vi "Channels.Inline.Block Data Ref to Descriptor.vi"(8 "error in (no error)":errorcluster, 11 "Block Data Ref":T3[](array[typedef]) {"Data Reference" format="%.0x"}) -> (0 "error out":errorcluster, 3 "Channel Block Descriptor":T1[](array[typedef]))   [LabVIEW 2016, in "VeriStand Data.lvlib"]
doc: "Converts a VeriStand <B>Block Data Ref</B> into a <B>Channel Block Descriptor</B> to allow for direct access of channel data."
uses:
  VeriStand Data.lvlib
  <vilib>/NI Veristand/Custom Device API/Block Data Reference.ctl
  <vilib>/NI Veristand/Custom Device API/Data Reference.ctl
  Typedefs/Typedefs.Block Descriptor.Channel Block.ctl
  Typedefs/Typedefs.Block Descriptor.ctl
  Channels.Inline.Data Reference to Pointer.vi
  Channels.Inline.Reference Error Handler.vi
  <vilib>/NI Veristand/Custom Device API/Global Data Refs.vi
  <vilib>/NI Veristand/Custom Device API/Custom Device API.lvlib
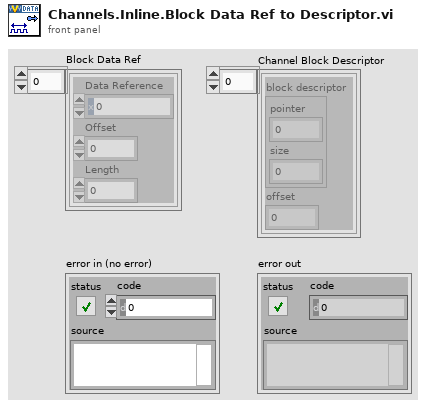
[diagram p1: front panel]
types:
  T1 = typedef "VeriStand Data.lvlib/Typedefs.Block Descriptor.Channel Block.ctl" = cluster{"block descriptor":T2, "offset":u64}
  T2 = typedef "VeriStand Data.lvlib/Typedefs.Block Descriptor.ctl" = cluster{"pointer":u64, "size":u64}
  T3 = typedef "Custom Device API.lvlib/Block Data Reference.ctl" = cluster{"Data Reference":T4, "Offset":u64, "Length":u64}
  T4 = typedef "Custom Device API.lvlib/Data Reference.ctl" = i32
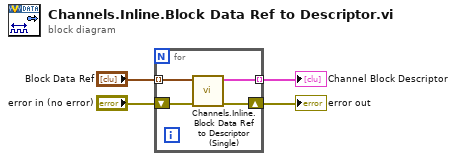
[diagram p0: block diagram]
diagram:
  n1 = for {
    tunnel: "Block Data Ref" -> [w8] mode=indexing
    tunnel: [w7] -> w3 mode=indexing
    shift-right: [w6] -> w1
    shift-left: "error in (no error)" -> [w5]
    n2 = call "Channels.Inline.Block Data Ref to Descriptor (Single).vi"("error in (no error)"=w5, "Block Data Ref"=w8) -> ("error out"=w6:errorcluster, "Channel Block Descriptor"=w7:T1)  [unwired: 8 in]
  }
  "Channel Block Descriptor" <- w3
  "error out" <- w1
